vi "Configure Multi Eval Meas Modulation EVM Window Length Selected BW.vi"(4 "Extended 60 kHz Spacing (0)":i32, 5 "Normal 60 kHz Spacing (0)":i32, 6 "Normal 30 kHz Spacing (0)":i32, 7 "Normal 15 kHz Spacing (0)":i32, 8 "error in (no error)":errorcluster, 9 "Bandwidth (5 MHz)":i32(ring)=5 items=["5 MHz"=5, "10 MHz"=10, "15 MHz"=15, "20 MHz"=20, "25 MHz"=25, "30 MHz"=30, "40 MHz"=40, "50 MHz"=50, "60 MHz"=60, "80 MHz"=80, "90 MHz"=90, "100 MHz"=100], 10 "Instance (1)":T1=1, 11 "VISA resource name":refnum<visa-resource-name>) -> (0 "error out":errorcluster, 3 "VISA resource name out":refnum<visa-resource-name>)   [LabVIEW 2020, in "Rohde&Schwarz CMWXP NR FR1 Measurement.lvlib"]
doc: "Specifies the EVM window length in samples for a selected channel bandwidth, depending on the SC spacing.\n\nAttribute:\nRSCMWXPNRFR1M_ATTR_MULTI_EVAL_MEAS_MODULATION_EVM_WINDOW_LENGTH_SELECTED_BW\n\nRemote-control command:\nCONFigure:NRSub:MEAS<i>:MEValuation:MODulation:EWLength:CBANdwidth<bw>"
uses:
  <instrlib>/Rohde&Schwarz CMWXP NR FR1 Measurement/Rohde&Schwarz CMWXP NR FR1 Measurement.lvlib
  <instrlib>/Rohde&Schwarz CMWXP NR FR1 Measurement/Private/_Instance.ctl
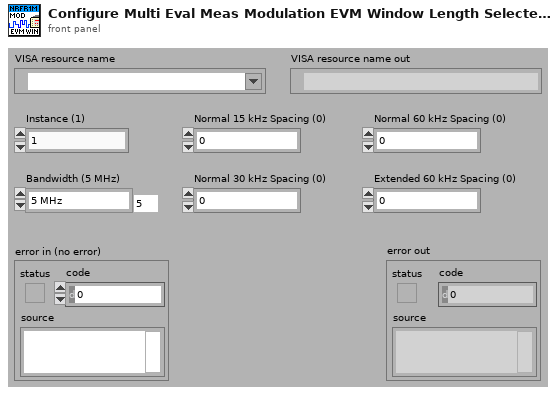
[diagram p1: front panel]
types:
  T1 = typedef "Rohde&Schwarz CMWXP NR FR1 Measurement.lvlib/_Instance.ctl" = i32
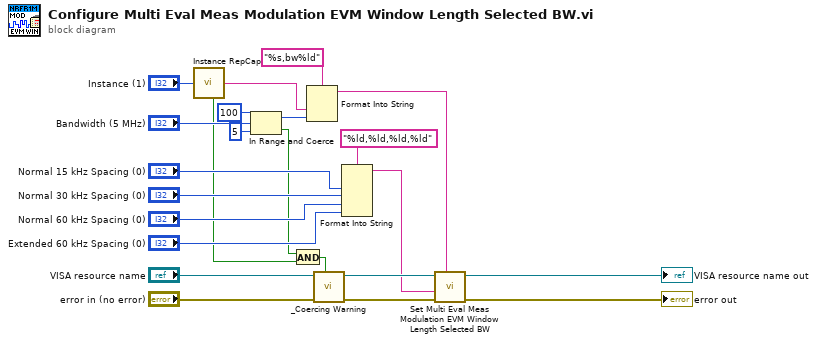
[diagram p0: block diagram]
diagram:
  n1 = call <instrlib>:"Instance RepCap.vi"("Instance In"="Instance (1)") -> ("In Range?"=w1:bool, "RepCap Identifier Out"=w18:string)  [unwired: 1 in]
  n2 = In Range and Coerce(upper limit=100, x="Bandwidth (5 MHz)", lower limit=5) -> (coerced(x)=w17:i32, In Range?=w3:bool)
  n3 = And(x=w3, y=w1) -> (x .and. y?=w2:bool)
  n4 = Format Into String(format string="%s,bw%ld", w18, w17) -> (resulting string=w10:string)  [unwired: 2 in, 1 out]
  n5 = call <instrlib>:"_Coercing Warning.vi"("In Range?"=w2, "error in (no error)"="error in (no error)", "VISA resource name"="VISA resource name") -> ("error out"=w14:errorcluster, "VISA resource name out"=w11:refnum<visa-resource-name>)  [unwired: 7 in]
  n6 = Format Into String(format string="%ld,%ld,%ld,%ld", "Normal 15 kHz Spacing (0)", "Normal 30 kHz Spacing (0)", "Normal 60 kHz Spacing (0)", "Extended 60 kHz Spacing (0)") -> (resulting string=w4:string)  [unwired: 2 in, 1 out]
  n7 = call "Set Multi Eval Meas Modulation EVM Window Length Selected BW"("Repeated Capabilities"=w10, "error in (no error)"=w14, "Multi Eval Meas Modulation EVM Window Length Selected BW ()"=w4, "instrument handle"=w11) -> ("error out"=→"error out":errorcluster, "instrument handle out"=→"VISA resource name out":refnum<visa-resource-name>)  [unwired: 6 in]
